vi "hSoftReset2013.vi"(4 "error in":errorcluster, 7 "FPGA VI Reference In":refnum<k20>) -> (0 "error out":errorcluster, 3 "FPGA VI Reference Out":refnum<k20>)   [LabVIEW 2014]
doc: "Gibt Reset-Impuls aus und setzt wichtige Elemente auf Ausgangszustand zurück."
uses:
  <vilib>/Utility/error.llb/Error Cluster From Error Code.vi
  <vilib>/rvi/errors/niLvFpgaAdjustHostInterfaceError.vi
  <vilib>/rvi/interface/nirviReadWriteControl/nirviReadWriteControl.xnode
  FPGA Bitfiles/W7XBolo2017_FPGATarget_FlorianDefault.lvbitx
  f_main_2014.vi
  NiFpgaLv.dll
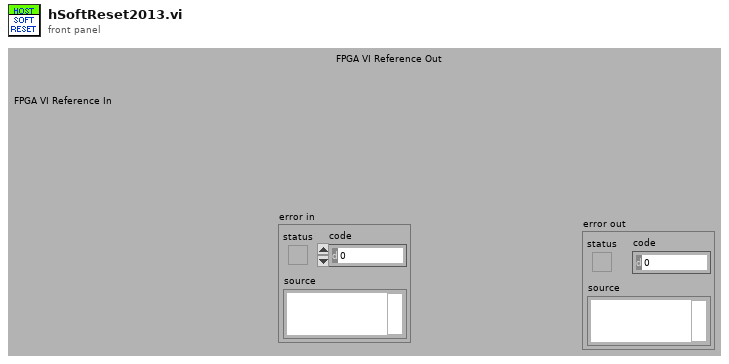
[diagram p1: front panel]
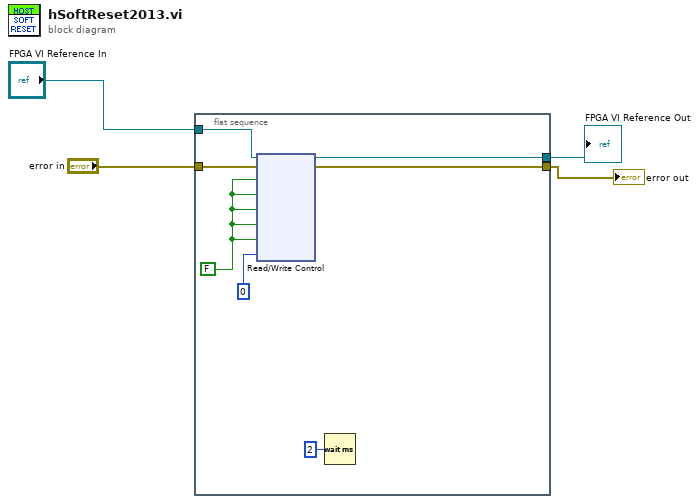
[diagram p0: block diagram]
diagram:
  n1 = flat-sequence {
    tunnel: "error in" -> [w8]
    tunnel: "FPGA VI Reference In" -> [w7]
    tunnel: [w6] -> w2
    tunnel: [w5] -> w3
    frame #0 {
      w10 = FALSE
      n2 = xnode "Read/Write Control"("FPGA VI Reference In"=w7, "error in"=w8, "Sprung0"=w10, "Sprung1"=w10, "HIREF"=w10, "RLY1"=w10, "RLY2"=w10, "ScanID"=u32 0 ("Comm ID")) -> ("FPGA VI Reference Out"=w6:refnum<k20>, "error out"=w5:errorcluster)
      n3 = Wait (ms)(milliseconds to wait=u16 2 ("Count(uSec)")) -> ()  [unwired: 1 out]
    }
  }
  "error out" <- w3
  "FPGA VI Reference Out" <- w2
